vi "Check for Included Angle.vi"   [LabVIEW 2020, in "NI_AAL_Angle.lvlib"]
doc: "Checks whether one or multiple input angles are within the counterclockwise range.\n\nWire data to any of the angle inputs to determine the polymorphic instance to use or manually select the instance."
uses:
  <vilib>/Analysis/NI_AAL_Angle.lvlib
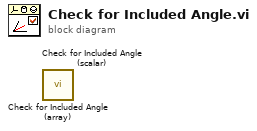
[diagram p0: block diagram]
diagram:
  n1 = call <vilib>:"Check for Included Angle (array).vi"() -> ()  [unwired: 9 in, 3 out]
  n2 = call <vilib>:"Check for Included Angle (scalar).vi"() -> ()  [unwired: 9 in, 3 out]
